vi "Parallel loops.vi"() -> ()   [LabVIEW 2014]
panel:
  in  "stop":bool
  out "Loop 2 executed":bool
  out "Loop 1 executed":bool
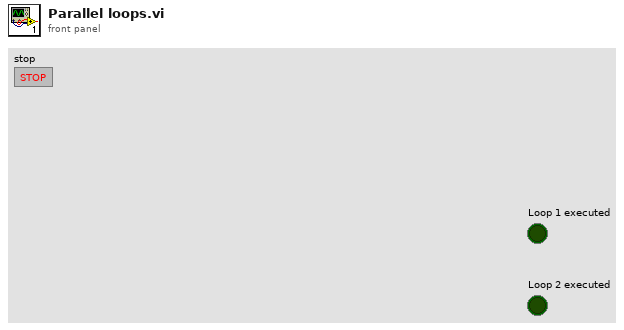
[diagram p1: front panel]
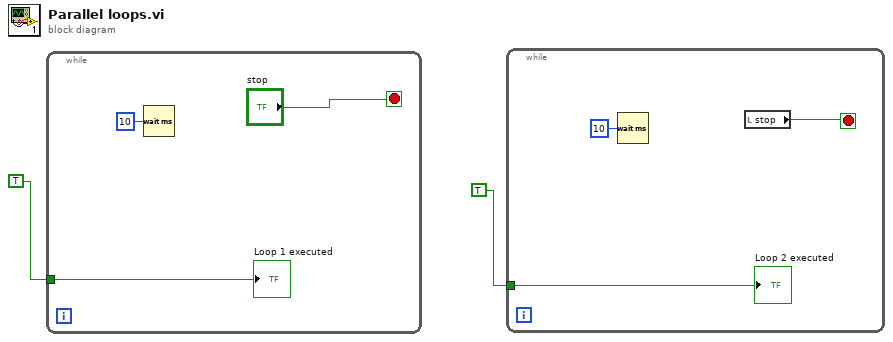
[diagram p0: block diagram]
diagram:
  n1 = while {
    tunnel: TRUE -> [w4]
    stop <- "stop" stop-if-true
    n2 = Wait (ms)(milliseconds to wait=u32 10) -> ()  [unwired: 1 out]
    "Loop 1 executed" <- w4
  }
  n3 = while {
    tunnel: TRUE -> [w7]
    stop <- w6 stop-if-true
    n4 = Wait (ms)(milliseconds to wait=u32 10) -> ()  [unwired: 1 out]
    n5 = local read "stop"() -> (w6:bool)
    "Loop 2 executed" <- w7
  }
